vi "PH_Cont-601k_PSU.Set Expert Mode.vi"(0 "VI in":refnum<vi>, 2 "Expert working":bool, 5 "error in (no error)":errorcluster) -> (14 "VI out":refnum<vi>, 19 "error out":errorcluster)   [LabVIEW 2014, in "PH_Cont-601k_PSU.lvlib"]
uses:
  PH_Cont-601k_PSU.lvlib
  PH_Cont-601k_PSU.Readyness Device.ctl
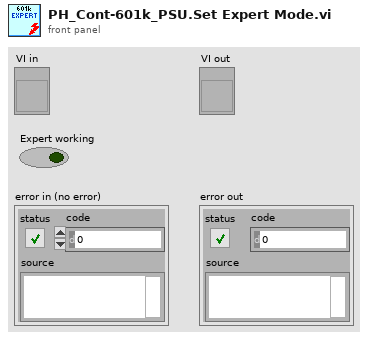
[diagram p1: front panel]
types:
  T1 = typedef "PH_Cont-601k_PSU.lvlib/PH_Cont-601k_PSU.Readyness Device.ctl" = enum32{"OFF", "CONNECTING", "CONNECTED", "OPERATING", "EOC", "ERROR"}
  T2 = enum8{"Enabled", "Disabled", "Disabled and Grayed Out"}
  T3 = typedef "PH_Cont-601k_PSU.lvlib/PH_Cont-601k_PSU.i attribute.ctl" = cluster{"GUI Refs":T4, "Interlock":bool, "Service ID applied Voltage":i32, "Device Settings":cluster{"Configuration":T5, "Flash Interval [s]":dbl, "Mode":T6, "Voltage [V]":u16, "Charge":bool, "VISA resource name":refnum<visa-resource-name>}, "Readyness":T7, "Information":cluster{"VISA resource name":refnum<visa-resource-name>, "Tagname Power On":string, "Interlock":cluster{"Instance":string, "Tagname":string}, "Limits [V]":cluster{"Lower":dbl, "Upper":dbl}, "Tagname PSU On":string}, "R2S":bool, "Charge is allowed":bool}
  T4 = typedef "PH_Cont-601k_PSU.lvlib/PH_Cont-601k_PSU.GUI Refs.ctl" = cluster{"Power On":refnum<vi>, "Hard- and Software":refnum<vi>, "Device Status":refnum<vi>, "Device Error":refnum<vi>, "Configuration":refnum<vi>, "Flash Interval [s]":refnum<vi>, "Interlock":refnum<vi>, "Interlock Indicator":refnum<vi>, "Voltage [V]":refnum<vi>, "Readyness":refnum<vi>, "Mode":refnum<vi>, "Reset Error":refnum<vi>, "Expert working":refnum<vi>, "Charge":refnum<vi>, "PSU On":refnum<vi>}
  T5 = typedef "PH_Cont-601k_PSU.lvlib/PH_Cont-601k_PSU.Configuration.ctl" = u16
  T6 = typedef "PH_Cont-601k_PSU.lvlib/PH_Cont-601k_PSU.Mode.ctl" = enum32{"STOP", "STANDBY", "READY", "EMISSION", "ERROR"}
  T7 = typedef "PH_Cont-601k_PSU.lvlib/PH_Cont-601k_PSU.Readyness.ctl" = cluster{"Program":T8, "Device":T1}
  T8 = typedef "PH_Cont-601k_PSU.lvlib/PH_Cont-601k_PSU.Readyness Program.ctl" = enum32{"OFF", "POWER", "INTERLOCK"}
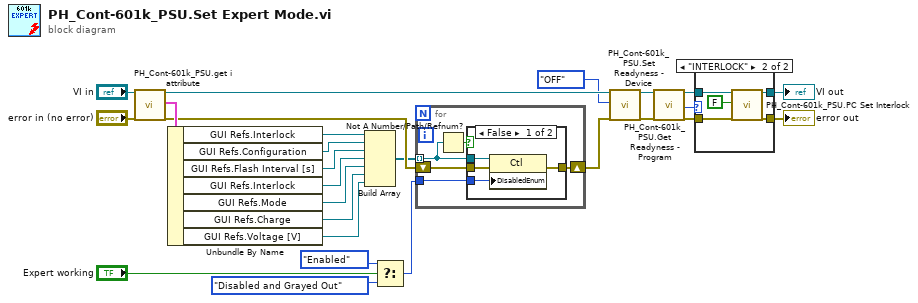
[diagram p0: block diagram]
diagram:
  n1 = call "PH_Cont-601k_PSU.get i attribute.vi"("i ref in"="VI in", "error in (no error)"="error in (no error)") -> ("i ref out"=w24:refnum<vi>, "i attribute"=w26:T3, "error out"=w25:errorcluster)  [unwired: 15 in]
  n2 = Unbundle By Name(w26) -> ("GUI Refs.Interlock"=w21:refnum<vi>, "GUI Refs.Configuration"=w20:refnum<vi>, "GUI Refs.Flash Interval [s]"=w19:refnum<vi>, "GUI Refs.Interlock"=w18:refnum<vi>, "GUI Refs.Mode"=w17:refnum<vi>, "GUI Refs.Charge"=w16:refnum<vi>, "GUI Refs.Voltage [V]"=w15:refnum<vi>)
  n3 = Build Array(w21, w20, w19, w18, w17, w16, w15) -> (w14:refnum<vi>[])
  n4 = Select(t=T2."Enabled" ("Disabled"), s="Expert working", f=T2."Disabled and Grayed Out") -> (s? t:f=w11:T2)
  n5 = for {
    tunnel: w14 -> [w29] mode=indexing
    shift-right: [w30] -> w9
    shift-left: w25 -> [w31]
    tunnel: w11 -> [w27]
    n6 = Not A Number/Path/Refnum?(number/path/refnum=w29) -> (NaN/Path/Refnum?=w28:bool)
    n7 = case shown="False" w28 {
      tunnel: w31 -> [w35 w36]
      tunnel: [w34 w36] -> w30
      tunnel: w29 -> [w33 _]
      tunnel: w27 -> [w32 _]
      frame False {
        n8 = property class="Ctl"(reference=w33, error in=w35, "DisabledEnum"=w32) -> (error out=w34:errorcluster)  [unwired: 1 out]
      }
      frame True {
      }
    }
  }
  n9 = call "PH_Cont-601k_PSU.Set Readyness - Device.vi"("VI in"=w24, "Readyness - Device"=PH_Cont-601k_PSU.Readyness_Device."OFF", "error in (no error)"=w9) -> ("VI out"=w7:refnum<vi>, "error out"=w6:errorcluster)  [unwired: 15 in]
  n10 = call "PH_Cont-601k_PSU.Get Readyness - Program.vi"("VI in"=w7, "error in (no error)"=w6) -> ("VI out"=w5:refnum<vi>, "Readyness - Programm"=w1:T8, "error out"=w4:errorcluster)  [unwired: 15 in]
  n11 = case shown="\"INTERLOCK\"" w1 {
    tunnel: w5 -> [w38 w43]
    tunnel: w4 -> [w37 w42]
    tunnel: [w37 w41] -> w3
    tunnel: [w38 w40] -> w2
    frame Default {
    }
    frame "INTERLOCK" {
      n12 = call "PH_Cont-601k_PSU.PC Set Interlock.vi"("VI in"=w43, "Set Interlock"=FALSE, "error in (no error)"=w42) -> ("VI out"=w40:refnum<vi>, "error out"=w41:errorcluster)  [unwired: 15 in]
    }
  }
  "error out" <- w3
  "VI out" <- w2
